vi "odchyl_stand_sub.vi"(0 "próbka":dbl[](array[numeric])) -> (1 "odchyl":dbl, 2 "œrednia":dbl)   [LabVIEW 2012]
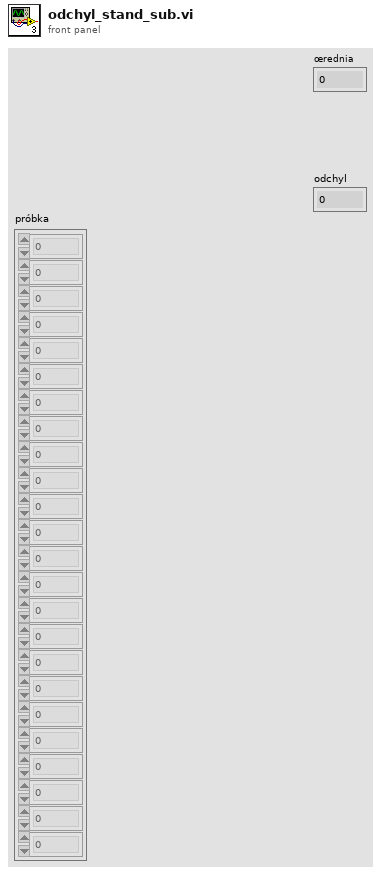
[diagram p1: front panel]
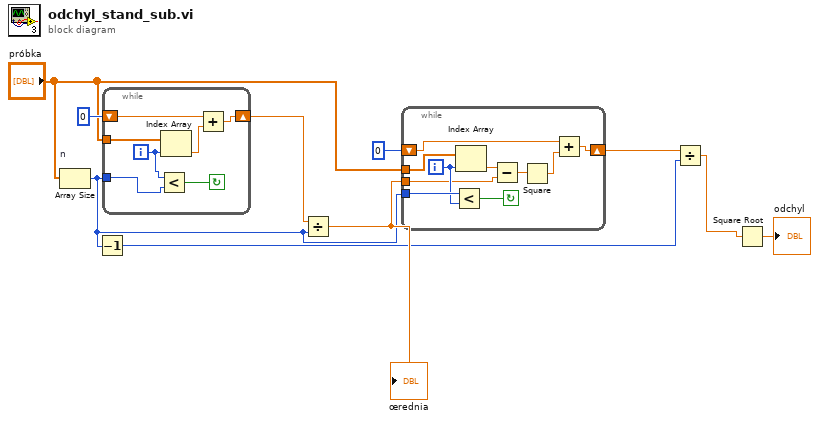
[diagram p0: block diagram]
diagram:
  n1 = Array Size "n"(array="próbka") -> (size(s)=w4:i32)
  n2 = Decrement(x=w4) -> (x-1=w2:i32)
  n3 = while {
    tunnel: "próbka" -> [w16]
    tunnel: w4 -> [w12]
    shift-right: [w13] -> w9
    shift-left: 0 -> [w15]
    i -> [w11]
    stop <- w17 continue-if-true
    n4 = Less?(x=w11, y=w12) -> (x < y?=w17:bool)
    n5 = Index Array(array=w16, index=w11) -> (element=w14:dbl)
    n6 = Add(x=w15, y=w14) -> (x+y=w13:dbl)
  }
  n7 = Divide(x=w9, y=w4) -> (x/y=w6:dbl)
  "œrednia" <- w6
  n8 = while {
    tunnel: "próbka" -> [w25]
    tunnel: w4 -> [w27]
    shift-right: [w22] -> w5
    shift-left: 0 -> [w23]
    tunnel: w6 -> [w20]
    i -> [w24]
    stop <- w26 continue-if-true
    n9 = Less?(x=w27, y=w24) -> (x < y?=w26:bool)
    n10 = Index Array(array=w25, index=w24) -> (element=w21:dbl)
    n11 = Subtract(x=w21, y=w20) -> (x-y=w19:dbl)
    n12 = Square(x=w19) -> (x^2=w18:dbl)
    n13 = Add(x=w23, y=w18) -> (x+y=w22:dbl)
  }
  n14 = Divide(x=w5, y=w2) -> (x/y=w1:dbl)
  n15 = Square Root(x=w1) -> (sqrt(x)=→"odchyl":dbl)
